vi "sendInfoToHost.vi"(11 "scan info":T1) -> (3 "ready for input":bool)   [LabVIEW 2010]
uses:
  <vilib>/rvi/DataTransferAndStorage/Container/XNode/niFpgaContainer.xnode
  <vilib>/rvi/DataTransferAndStorage/Container/Common/niFpgaContainerMethod.ctl
  <vilib>/rvi/DataTransferAndStorage/Container/Common/niFpgaTransferTypeControl.ctl
  <vilib>/rvi/interface/RandomDataEmulation/nirviRandomDataFPGAFIFO.vi
  <vilib>/rvi/interface/RandomDataEmulation/niFpgaRandomDataHandleErrors.vi
panel:
  out "command lost":bool
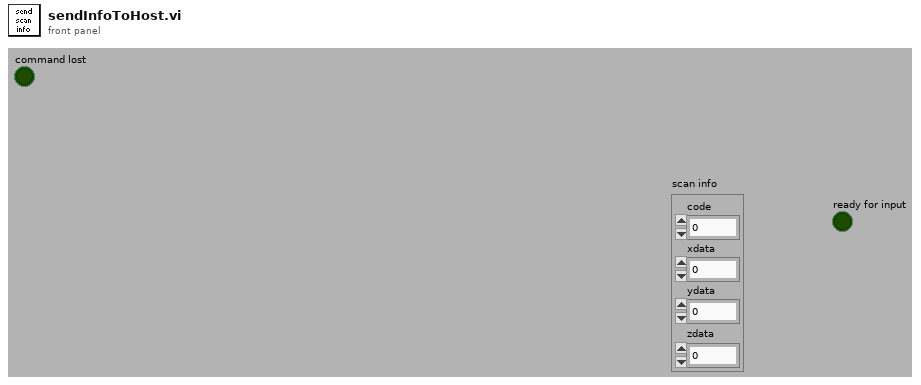
[diagram p1: front panel]
types:
  T1 = cluster{"code":i32, "xdata":i32, "ydata":i32, "zdata":i32}
  T2 = enum16{"NONE", "VOLUME_START", "LINE_START", "LINE_END", "VOLUME_END"}
  T3 = typedef "niFpgaContainerMethod.ctl" = enum16{"<none>", "write", "read", "clear", "getNumberOfElementsToWrite", "getNumberOfElementsToRead", "enable", "disable", "flushAndDisable", "getStreamState", "readA", "readB", "dramWrite", "dramWriteWithByteEnables", "dramRequestData", "dramRetrieveData"}
  T4 = typedef "niFpgaTransferTypeControl.ctl" = enum16{"Target-Scoped", "Host to Target - DMA", "Target to Host - DMA", "Peer to Peer Reader", "Peer to Peer Writer", "Bidirectional"}
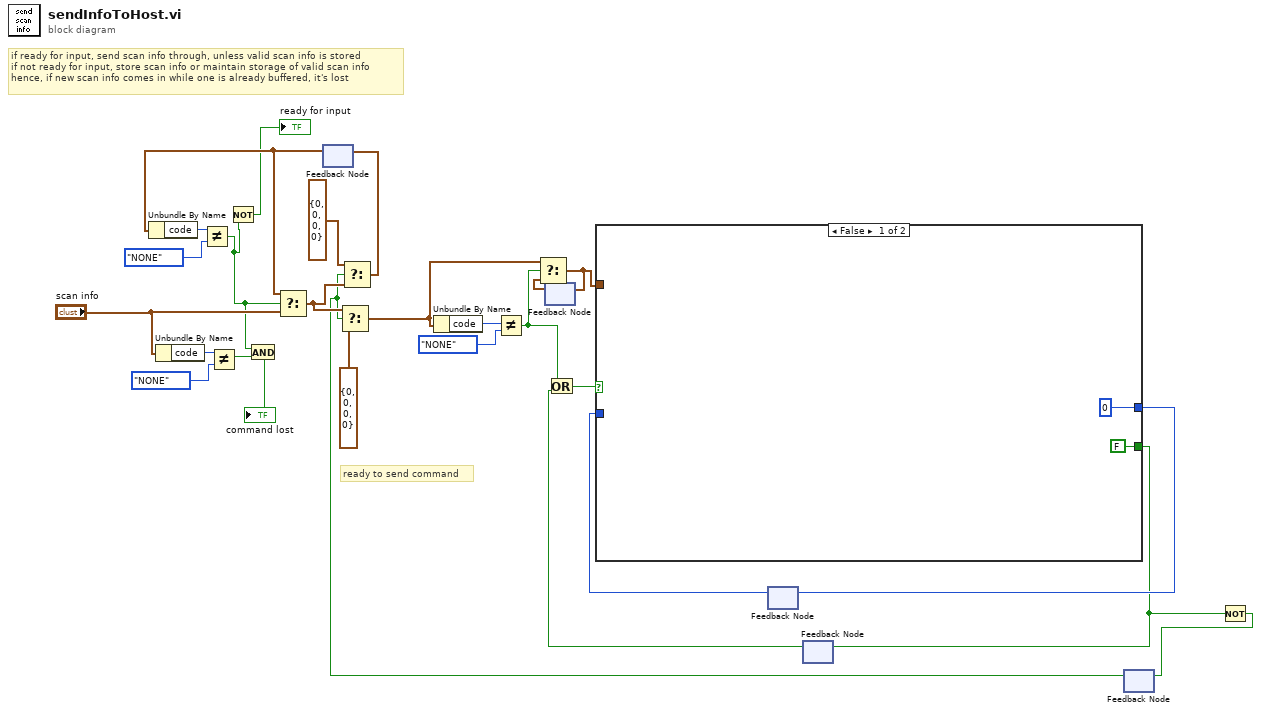
[diagram p0: block diagram]
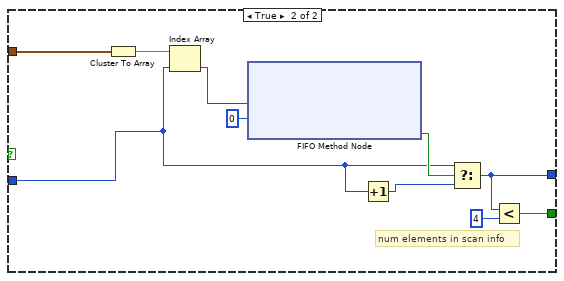
[diagram p2: hidden frame]
diagram:
  # "ready to send command"
  # "if ready for input, send scan info through, unless valid scan info is stored\nif not ready for input, store scan info or maintain storage of valid scan info\nhence, if new scan info comes in while one is already buffered, it's lost"
  n1 = Unbundle By Name("scan info") -> ("code"=w10:i32)
  n2 = Not Equal?(x=w10, y=T2."NONE" ("message")) -> (x != y?=w8:bool)
  n3 = feedback #1() -> (w11:T1)  [unwired: 1 in]
  n4 = Unbundle By Name(w11) -> ("code"=w17:i32)
  n5 = Not Equal?(x=w17, y=T2."NONE" ("message")) -> (x != y?=w3:bool)
  n6 = Not(x=w3) -> (.not. x?=→"ready for input":bool)
  n7 = And(x=w3, y=w8) -> (x .and. y?=→"command lost":bool)
  n8 = Select(t=w11, s=w3, f="scan info") -> (s? t:f=w14:T1)
  n9 = feedback #2() -> (w23:T1)  [unwired: 1 in]
  n10 = feedback #3() -> (w25:i32)  [unwired: 1 in]
  n11 = feedback #4() -> (w24:bool)  [unwired: 1 in]
  n12 = feedback #5() -> (w1:bool)  [unwired: 1 in]
  n13 = Select(t=w14, s=w1, f=T1 {"code"=0, "xdata"=0, "ydata"=0, "zdata"=0} ("scan info")) -> (s? t:f=w5:T1)
  n14 = Select(t=T1 {"code"=0, "xdata"=0, "ydata"=0, "zdata"=0} ("scan info"), s=w1, f=w14) -> (s? t:f=w12:T1)
  n15 = feedback-in #1(w12) -> ()
  n16 = Unbundle By Name(w5) -> ("code"=w21:i32)
  n17 = Not Equal?(x=w21, y=T2."NONE" ("message")) -> (x != y?=w18:bool)
  n18 = Select(t=w5, s=w18, f=w23) -> (s? t:f=w22:T1)
  n19 = feedback-in #2(w22) -> ()
  n20 = Or(x=w18, y=w24) -> (x .or. y?=w27:bool)
  n21 = case shown="False" w27 {
    tunnel: [0 ("index") w33] -> w26
    tunnel: w25 -> [_ w34]
    tunnel: [FALSE w31] -> w19
    tunnel: w22 -> [_ w30]
    frame False {
    }
    frame True {
      # "num elements in scan info"
      n22 = Cluster To Array(cluster=w30) -> (array=w39:i32[])
      n23 = Index Array(array=w39, index=w34) -> (element=w38:i32)
      n24 = xnode ("FIFO Method Node")("Element"=w38, "Timeout"=0) -> ("Timed Out?"=w36:bool)  [unwired: 1 in, 1 out]
      n25 = Increment(x=w34) -> (x+1=w35:i32)
      n26 = Select(t=w34, s=w36, f=w35) -> (s? t:f=w33:i32)
      n27 = Less?(x=w33, y=4) -> (x < y?=w31:bool)
    }
  }
  n28 = feedback-in #3(w26) -> ()
  n29 = feedback-in #4(w19) -> ()
  n30 = Not(x=w19) -> (.not. x?=w4:bool)
  n31 = feedback-in #5(w4) -> ()
